vi "Air Poker Top.vi.vi"() -> ()   [LabVIEW 2014]
uses:
  Card Used array.vi
  Global Hint.vi
panel:
  in  "Function Cluster":cluster{"Hint":bool, "Rule":bool, "About":bool}
  out "Card used array":dbl[](array[numeric])
  out "Round":i32
  out "B's Random Number":i32
  out "B's 5 Card array":i32[](array[numeric])
  out "A's Random Number":i32
  out "A's 5 Card array":i32[](array[numeric])
  in  "Start":bool
  out "Player B":T1(array[cluster])
  out "Player A":T1(array[cluster])
  out "Winner":string
  in  "Cluster":T2
  in  "Show Result":bool
  in  "End Game":bool
  in  "Next Round":bool
  # "Long press"
  # "Click here to watch other combinations"
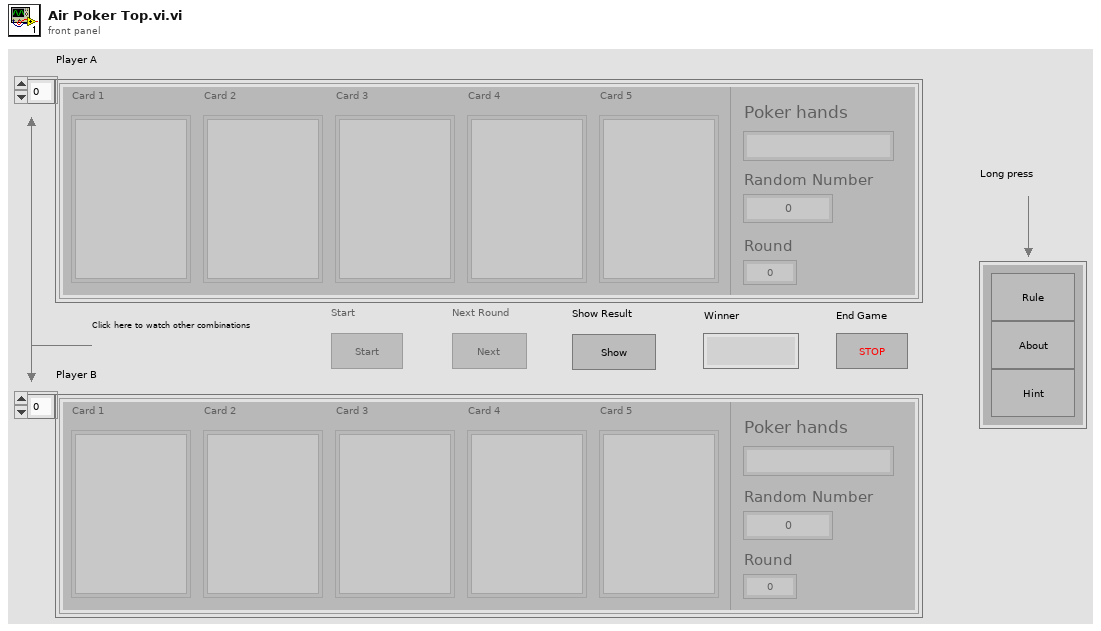
[diagram p1: front panel]
types:
  T1 = cluster{"Cluster 2":cluster{"Card 1":u16, "Card 2":u16, "Card 3":u16, "Card 4":u16, "Card 5":u16}, "Poker hands":string, "Random Number":dbl, "Round":i32}[]
  T2 = cluster{"element":dbl, "element":dbl, "element":dbl, "element":dbl, "element":dbl}
  T3 = enum8{"Enabled", "Disabled", "Disabled and Grayed Out"}
  T4 = cluster{"Cluster":cluster{"element":dbl, "element":dbl, "element":dbl, "element":dbl, "element":dbl}, string, "B's Random Number":i32, "Round":i32}
  T5 = cluster{"Cluster":cluster{"element":dbl, "element":dbl, "element":dbl, "element":dbl, "element":dbl}, string, "A's Random Number":i32, "Round":i32}
  T6 = cluster{"Score":dbl, cluster{"Rank":i32, cluster{"element":dbl, "element":dbl, "element":dbl, "element":dbl, "element":dbl}, "Poker hands":string}}[]
  T7 = cluster{"Rank":i32, cluster{"element":dbl, "element":dbl, "element":dbl, "element":dbl, "element":dbl}, "Poker hands":string}
  T8 = cluster{"Poker output":dbl, "Poker output 2":dbl, "Poker output 3":dbl, "Poker output 4":dbl, "Poker output 5":dbl}
  T9 = cluster{cluster{"Poker output":dbl, "Poker output 2":dbl, "Poker output 3":dbl, "Poker output 4":dbl, "Poker output 5":dbl}, "Poker hands":string, "A's Random Number":i32, "Round":i32}
  T10 = cluster{cluster{"Poker output":dbl, "Poker output 2":dbl, "Poker output 3":dbl, "Poker output 4":dbl, "Poker output 5":dbl}, "Poker hands":string, "B's Random Number":i32, "Round":i32}
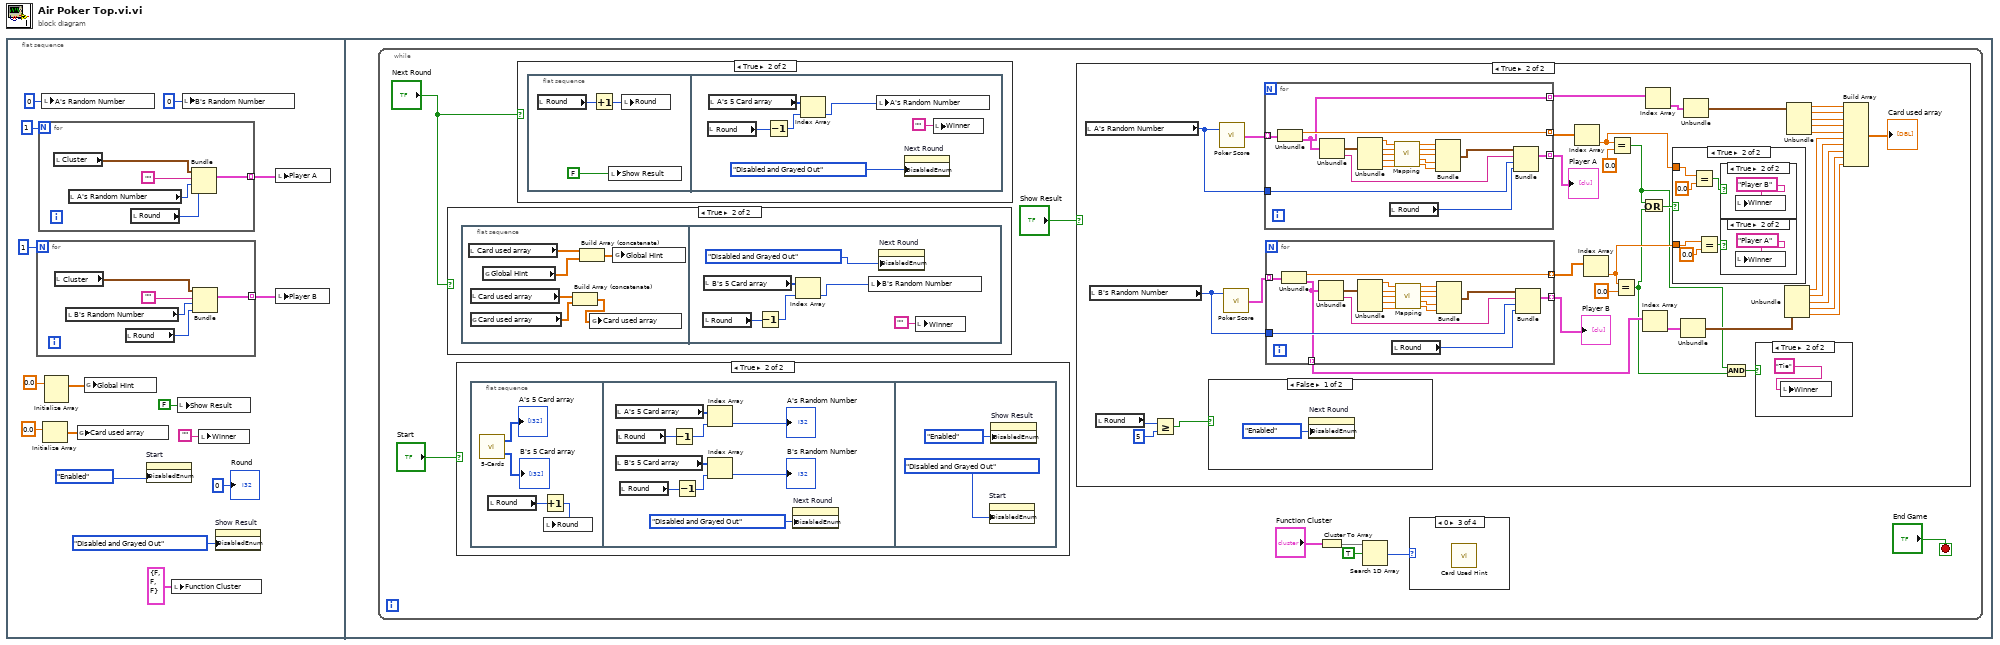
[diagram p0: block diagram]
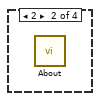
[diagram p3: hidden frame]
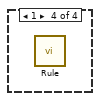
[diagram p4: hidden frame]
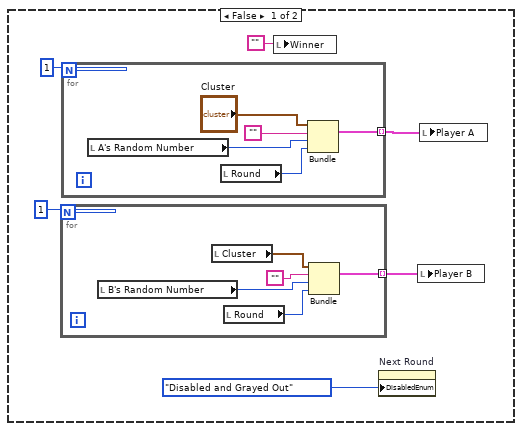
[diagram p7: hidden frame]
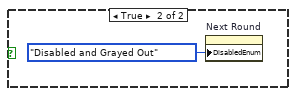
[diagram p8: hidden frame]
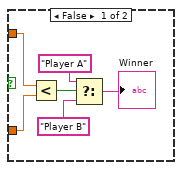
[diagram p10: hidden frame]
diagram:
  n1 = flat-sequence {
    frame #0 {
      n2 = for {
        N: 1 -> [_]
        tunnel: [w21] -> w9 mode=indexing
        n3 = local read "Cluster"() -> (w19:T2)
        n4 = local read "B's Random Number"() -> (w18:i32)
        n5 = local read "Round"() -> (w17:i32)
        n6 = Bundle("Cluster"=w19, "", "B's Random Number"=w18, "Round"=w17) -> (w21:T4)  [unwired: 1 in]
      }
      n7 = for {
        N: 1 -> [_]
        tunnel: [w26] -> w15 mode=indexing
        n8 = local read "Cluster"() -> (w24:T2)
        n9 = local read "A's Random Number"() -> (w23:i32)
        n10 = local read "Round"() -> (w22:i32)
        n11 = Bundle("Cluster"=w24, "", "A's Random Number"=w23, "Round"=w22) -> (w26:T5)  [unwired: 1 in]
      }
      n12 = local write "A's Random Number"(0 ("A's Random Number")) -> ()
      n13 = Initialize Array(0.0 ("element")) -> (w4:dbl[])  [unwired: 1 in]
      n14 = Initialize Array(0.0 ("element")) -> (w3:dbl[][])  [unwired: 2 in]
      n15 = global write "Card Used array.vi" "Card used array"(w4) -> ()
      n16 = global write "Global Hint.vi" "Global Hint"(w3) -> ()
      n17 = property on="Start" class="Bool"("DisabledEnum"=T3."Enabled" ("Disabled")) -> ()  [unwired: 2 in, 2 out]
      n18 = local write "Function Cluster"(cluster{"Hint":bool, "Rule":bool, "About":bool} {"Hint"=FALSE, "Rule"=FALSE, "About"=FALSE} ("Function Cluster")) -> ()
      n19 = local write "Show Result"(FALSE ("Show Result")) -> ()
      n20 = local write "B's Random Number"(0 ("A's Random Number")) -> ()
      n21 = local write "Winner"("") -> ()
      n22 = property on="Show Result" class="Bool (strict)"("DisabledEnum"=T3."Disabled and Grayed Out" ("Disabled")) -> ()  [unwired: 2 in, 2 out]
      n23 = local write "Player A"(w15) -> ()
      n24 = local write "Player B"(w9) -> ()
      "Round" <- 0 ("Round")
    }
    frame #1 {
      n25 = while {
        stop <- "End Game" stop-if-true
        n26 = case shown="True" "Next Round" {
          frame False {
          }
          frame True {
            n27 = flat-sequence {
              frame #0 {
                n28 = local read "Card used array"() -> (w35:dbl[])
                n29 = local read "Card used array"() -> (w40:dbl[])
                n30 = global read "Card Used array.vi" "Card used array"() -> (w39:dbl[])
                n31 = global read "Global Hint.vi" "Global Hint"() -> (w36:dbl[][])
                n32 = Build Array (concatenate)(w40, w39) -> (w38:dbl[])
                n33 = Build Array (concatenate)(w35, w36) -> (w37:dbl[][])
                n34 = global write "Card Used array.vi" "Card used array"(w38) -> ()
                n35 = global write "Global Hint.vi" "Global Hint"(w37) -> ()
              }
              frame #1 {
                n36 = local read "Round"() -> (w43:i32)
                n37 = local read "B's 5 Card array"() -> (w45:i32[])
                n38 = Decrement(x=w43) -> (x-1=w42:i32)
                n39 = Index Array(array=w45, index=w42) -> (element=w44:i32)
                n40 = local write "B's Random Number"(w44) -> ()
                n41 = property on="Next Round" class="Bool"("DisabledEnum"=T3."Disabled and Grayed Out" ("Disabled")) -> ()  [unwired: 2 in, 2 out]
                n42 = local write "Winner"("") -> ()
              }
            }
          }
        }
        n43 = case shown="True" "Start" {
          frame False {
          }
          frame True {
            n44 = flat-sequence {
              frame #0 {
                n45 = call "5-Cards.vi"() -> ("Array"=→"B's 5 Card array":i32[], "Array 2"=→"A's 5 Card array":i32[])  [unwired: 2 in]
                n46 = local read "Round"() -> (w50:i32)
                n47 = Increment(x=w50) -> (x+1=w49:i32)
                n48 = local write "Round"(w49) -> ()
              }
              frame #1 {
                n49 = local read "A's 5 Card array"() -> (w59:i32[])
                n50 = local read "B's 5 Card array"() -> (w56:i32[])
                n51 = local read "Round"() -> (w52:i32)
                n52 = local read "Round"() -> (w53:i32)
                n53 = Decrement(x=w52) -> (x-1=w51:i32)
                n54 = Decrement(x=w53) -> (x-1=w54:i32)
                n55 = Index Array(array=w59, index=w51) -> (element=→"A's Random Number":i32)
                n56 = Index Array(array=w56, index=w54) -> (element=→"B's Random Number":i32)
                n57 = property on="Next Round" class="Bool"("DisabledEnum"=T3."Disabled and Grayed Out" ("Disabled")) -> ()  [unwired: 2 in, 2 out]
              }
              frame #2 {
                n58 = property on="Start" class="Bool"("DisabledEnum"=T3."Disabled and Grayed Out" ("Disabled")) -> ()  [unwired: 2 in, 2 out]
                n59 = property on="Show Result" class="Bool (strict)"("DisabledEnum"=T3."Enabled" ("Disabled")) -> ()  [unwired: 2 in, 2 out]
              }
            }
          }
        }
        n60 = case shown="True" "Next Round" {
          frame False {
          }
          frame True {
            n61 = flat-sequence {
              frame #0 {
                n62 = local read "Round"() -> (w171:i32)
                n63 = Increment(x=w171) -> (x+1=w170:i32)
                n64 = local write "Show Result"(FALSE ("Show Result")) -> ()
                n65 = local write "Round"(w170) -> ()
              }
              frame #1 {
                n66 = local read "Round"() -> (w174:i32)
                n67 = local read "A's 5 Card array"() -> (w176:i32[])
                n68 = Decrement(x=w174) -> (x-1=w173:i32)
                n69 = Index Array(array=w176, index=w173) -> (element=w175:i32)
                n70 = local write "A's Random Number"(w175) -> ()
                n71 = property on="Next Round" class="Bool"("DisabledEnum"=T3."Disabled and Grayed Out" ("Disabled")) -> ()  [unwired: 2 in, 2 out]
                n72 = local write "Winner"("") -> ()
              }
            }
          }
        }
        n73 = case shown="True" "Show Result" {
          frame False {
            n74 = for {
              N: 1 -> [_]
              tunnel: [w72] -> w64 mode=indexing
              n75 = local read "B's Random Number"() -> (w69:i32)
              n76 = local read "Cluster"() -> (w70:T2)
              n77 = local read "Round"() -> (w68:i32)
              n78 = Bundle("Cluster"=w70, "", "B's Random Number"=w69, "Round"=w68) -> (w72:T4)  [unwired: 1 in]
            }
            n79 = for {
              N: 1 -> [_]
              tunnel: [w77] -> w63 mode=indexing
              n80 = local read "A's Random Number"() -> (w74:i32)
              n81 = local read "Round"() -> (w73:i32)
              n82 = Bundle("Cluster"="Cluster", "", "A's Random Number"=w74, "Round"=w73) -> (w77:T5)  [unwired: 1 in]
            }
            n83 = local write "Winner"("") -> ()
            n84 = property on="Next Round" class="Bool"("DisabledEnum"=T3."Disabled and Grayed Out" ("Disabled")) -> ()  [unwired: 2 in, 2 out]
            n85 = local write "Player B"(w64) -> ()
            n86 = local write "Player A"(w63) -> ()
          }
          frame True {
            n87 = local read "A's Random Number"() -> (w112:i32)
            n88 = local read "B's Random Number"() -> (w108:i32)
            n89 = local read "Round"() -> (w78:i32)
            n90 = Greater Or Equal?(x=w78, y=5) -> (x >= y?=w80:bool)
            n91 = case shown="False" w80 {
              frame False {
                n92 = property on="Next Round" class="Bool"("DisabledEnum"=T3."Enabled" ("Disabled")) -> ()  [unwired: 2 in, 2 out]
              }
              frame True {
                n93 = property on="Next Round" class="Bool"("DisabledEnum"=T3."Disabled and Grayed Out" ("Disabled")) -> ()  [unwired: 2 in, 2 out]
              }
            }
            n94 = call "Poker Score.vi"("Card Number"=w112) -> ("Poker Hands Score and Combination"=w111:T6)  [unwired: 1 in]
            n95 = call "Poker Score.vi"("Card Number"=w108) -> ("Poker Hands Score and Combination"=w110:T6)  [unwired: 1 in]
            n96 = for {
              tunnel: w111 -> [w168] mode=indexing
              tunnel: [w167] -> w107 mode=indexing
              tunnel: w112 -> [w166]
              tunnel: [w165] -> w113 mode=indexing
              tunnel: [w150] -> w103 mode=indexing
              n97 = Unbundle(w168) -> ("Score"=w165:dbl, w150:T7)
              n98 = Unbundle(w150) -> (w164:T2, "Poker hands"=w153:string)  [unwired: 1 out]
              n99 = Unbundle(w164) -> ("element"=w163:dbl, "element"=w162:dbl, "element"=w161:dbl, "element"=w160:dbl, "element"=w159:dbl)
              n100 = local read "Round"() -> (w151:i32)
              n101 = call "Mapping.vi"("DBL Input"=w163, "DBL Input 2"=w162, "DBL Input 3"=w161, "DBL Input 4"=w160, "DBL Input 5"=w159) -> ("Poker output"=w158:dbl, "Poker output 2"=w157:dbl, "Poker output 3"=w156:dbl, "Poker output 4"=w155:dbl, "Poker output 5"=w154:dbl)  [unwired: 6 in]
              n102 = Bundle("Poker output"=w158, "Poker output 2"=w157, "Poker output 3"=w156, "Poker output 4"=w155, "Poker output 5"=w154) -> (w152:T8)  [unwired: 1 in]
              n103 = Bundle(w152, "Poker hands"=w153, "A's Random Number"=w166, "Round"=w151) -> (w167:T9)  [unwired: 1 in]
            }
            "Player A" <- w107
            n104 = for {
              tunnel: w110 -> [w149] mode=indexing
              tunnel: [w148] -> w105 mode=indexing
              tunnel: [w147] -> w109 mode=indexing
              tunnel: w108 -> [w133]
              tunnel: [w131] -> w102 mode=indexing
              n105 = Unbundle(w149) -> ("Score"=w147:dbl, w131:T7)
              n106 = Unbundle(w131) -> (w146:T2, "Poker hands"=w134:string)  [unwired: 1 out]
              n107 = Unbundle(w146) -> ("element"=w145:dbl, "element"=w144:dbl, "element"=w143:dbl, "element"=w142:dbl, "element"=w141:dbl)
              n108 = local read "Round"() -> (w132:i32)
              n109 = call "Mapping.vi"("DBL Input"=w145, "DBL Input 2"=w144, "DBL Input 3"=w143, "DBL Input 4"=w142, "DBL Input 5"=w141) -> ("Poker output"=w140:dbl, "Poker output 2"=w139:dbl, "Poker output 3"=w138:dbl, "Poker output 4"=w137:dbl, "Poker output 5"=w136:dbl)  [unwired: 6 in]
              n110 = Bundle("Poker output"=w140, "Poker output 2"=w139, "Poker output 3"=w138, "Poker output 4"=w137, "Poker output 5"=w136) -> (w135:T8)  [unwired: 1 in]
              n111 = Bundle(w135, "Poker hands"=w134, "B's Random Number"=w133, "Round"=w132) -> (w148:T10)  [unwired: 1 in]
            }
            "Player B" <- w105
            n112 = Index Array(array=w113) -> (element=w85:dbl)  [unwired: 1 in]
            n113 = Index Array(array=w109) -> (element=w84:dbl)  [unwired: 1 in]
            n114 = Equal?(x=w85, y=0.0) -> (x = y?=w82:bool)
            n115 = Equal?(x=w84, y=0.0) -> (x = y?=w81:bool)
            n116 = Or(x=w82, y=w81) -> (x .or. y?=w86:bool)
            n117 = Index Array(array=w102) -> (element=w104:T7)  [unwired: 1 in]
            n118 = Index Array(array=w103) -> (element=w106:T7)  [unwired: 1 in]
            n119 = case shown="True" w86 {
              tunnel: w85 -> [w118 w128]
              tunnel: w84 -> [w117 w124]
              frame False {
                n120 = Less?(x=w118, y=w117) -> (x < y?=w119:bool)
                n121 = Select(t="Player A", s=w119, f="Player B") -> (s? t:f=→"Winner":string)
              }
              frame True {
                n122 = Equal?(x=w128, y=0.0) -> (x = y?=w126:bool)
                n123 = Equal?(x=w124, y=0.0) -> (x = y?=w123:bool)
                n124 = case shown="True" w126 {
                  frame False {
                  }
                  frame True {
                    n125 = local write "Winner"("Player B") -> ()
                  }
                }
                n126 = case shown="True" w123 {
                  frame False {
                  }
                  frame True {
                    n127 = local write "Winner"("Player A") -> ()
                  }
                }
              }
            }
            n128 = Unbundle(w104) -> (w95:T2)  [unwired: 2 out]
            n129 = Unbundle(w106) -> (w101:T2)  [unwired: 2 out]
            n130 = And(x=w82, y=w81) -> (x .and. y?=w83:bool)
            n131 = case shown="True" w83 {
              frame False {
              }
              frame True {
                n132 = local write "Winner"("Tie") -> ()
              }
            }
            n133 = Unbundle(w95) -> ("element"=w94:dbl, "element"=w93:dbl, "element"=w92:dbl, "element"=w91:dbl, "element"=w90:dbl)
            n134 = Unbundle(w101) -> ("element"=w100:dbl, "element"=w99:dbl, "element"=w98:dbl, "element"=w97:dbl, "element"=w96:dbl)
            n135 = Build Array(w100, w99, w98, w97, w96, w94, w93, w92, w91, w90) -> (→"Card used array":dbl[])
          }
        }
        n136 = Cluster To Array(cluster="Function Cluster") -> (array=w29:bool[])
        n137 = Search 1D Array(1D array=w29, element=TRUE) -> (index of element=w27:i32)  [unwired: 1 in]
        n138 = case shown="0" w27 {
          frame -1, Default {
          }
          frame 2 {
            n139 = call "About.vi"() -> ()  [unwired: 12 in]
          }
          frame 0 {
            n140 = call "Card Used Hint.vi"() -> ()  [unwired: 1 in, 1 out]
          }
          frame 1 {
            n141 = call "Rule.vi"() -> ()  [unwired: 12 in]
          }
        }
      }
    }
  }
